vi "SUB_BatterySW_Powff_Indicate.vi"(3 "String":string) -> ()   [LabVIEW 2011]
doc: "This is an example of how to use the radio buttons control with the Value Changed event."
panel:
  in  "電池開關往下推":bool
  out "EXIT 2":enum32{"No Selection", "EXIT", "None"}(ring)
  out "EXIT":enum32{"No Selection", "EXIT", "None"}(ring)
  in  "把電池開關往下推後.點選EXIT離開":enum32{"No Selection", "EXIT", "None"}(radio)=enum."EXIT"
  # "電池開關需往下推"
  # "注意事項\n1.Mobile 線需拔除\n\n2.電池開關需往下推"
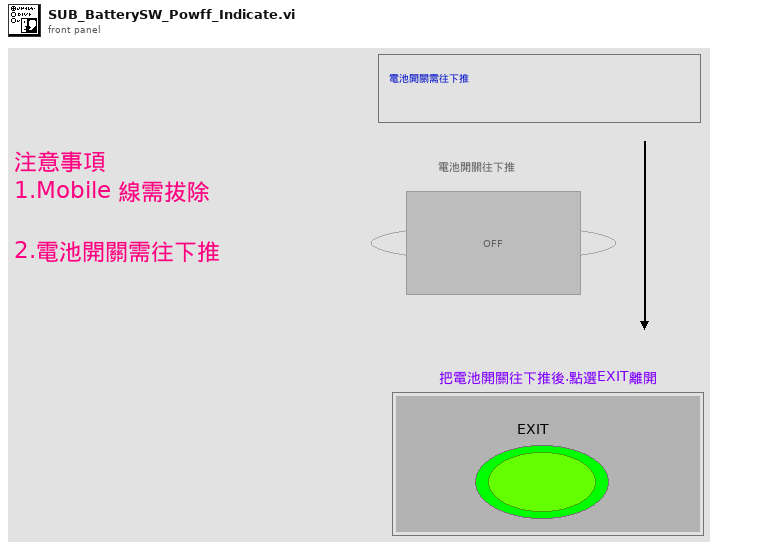
[diagram p1: front panel]
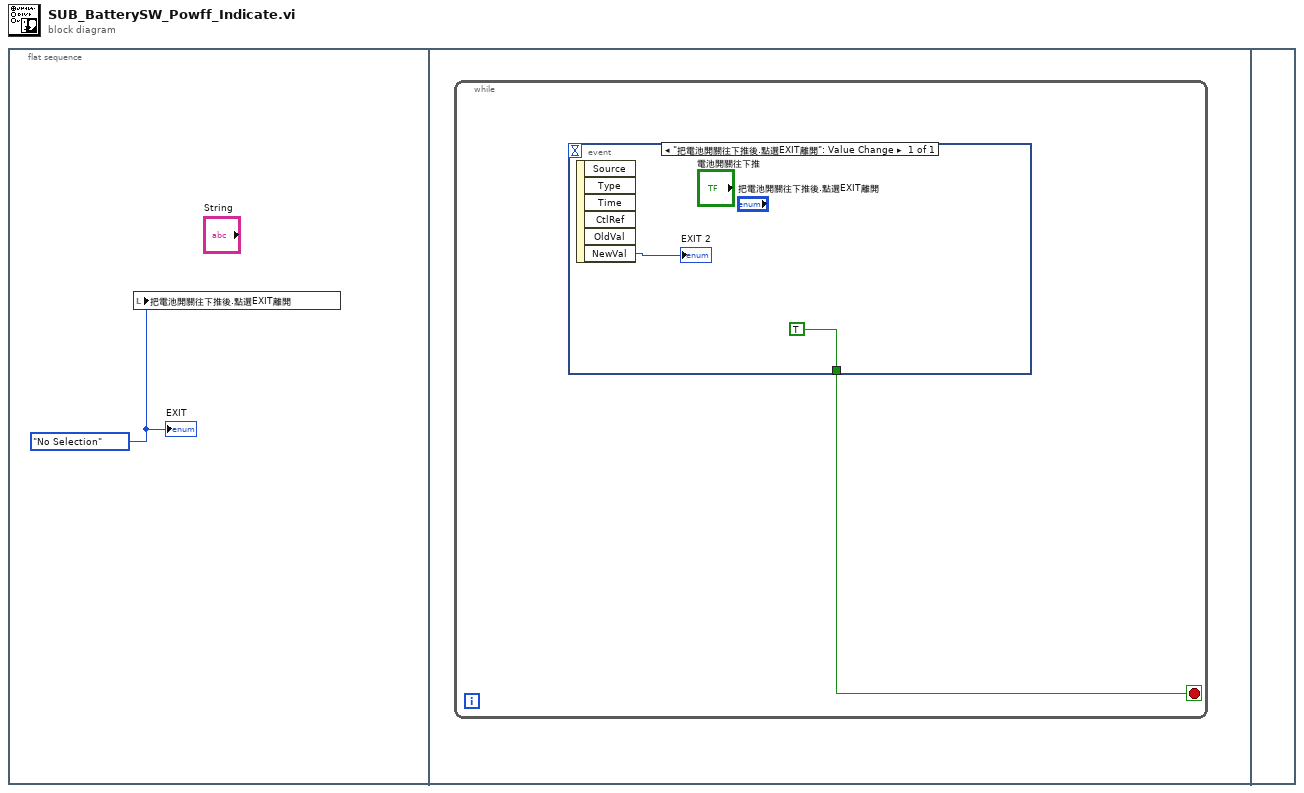
[diagram p0: block diagram]
diagram:
  n1 = flat-sequence {
    frame #0 {
      w1 = enum32{"No Selection", "EXIT", "None"}."No Selection" ("yes/no")
      n2 = local write "把電池開關往下推後.點選EXIT離開"(w1) -> ()
      "EXIT" <- w1
    }
    frame #1 {
      n3 = while {
        stop <- w2 stop-if-true
        n4 = event shown="[0] \"把電池開關往下推後.點選EXIT離開\": Value Change" {
          selector: _ -> [_]
          dyn-events: _ -> [_]
          timeout: _ -> [_]
          tunnel: [TRUE] -> w2
          event "把電池開關往下推後.點選EXIT離開": Value Change {
            n5 = event-data() -> ("NewVal"=→"EXIT 2":enum32{"No Selection", "EXIT", "None"})  [unwired: 1 in, 5 out]
          }
        }
      }
    }
    frame #2 {
    }
  }
